vi "Tnaught.vi"(11 "Ring":u16(ring) items=["Check", "Init"]) -> (3 "Numeric":dbl)   [LabVIEW 2019]
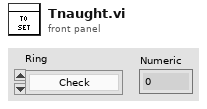
[diagram p1: front panel]
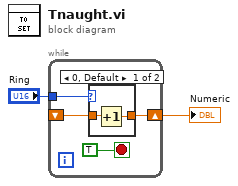
[diagram p0: block diagram]
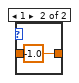
[diagram p2: hidden frame]
diagram:
  n1 = while {
    tunnel: "Ring" -> [w5]
    shift-right: [w3] -> w1
    shift-left: _ -> [w4]
    stop <- TRUE stop-if-true
    n2 = case shown="0, Default" w5 {
      tunnel: w4 -> [w8 _]
      tunnel: [w7 -1.0] -> w3
      frame 0, Default {
        n3 = Increment(x=w8) -> (x+1=w7:dbl)
      }
      frame 1 {
      }
    }
  }
  "Numeric" <- w1
